vi "sftp_rename.vi"() -> ()   [LabVIEW 2017]
doc: "Illustrates how to rename a file on an SSH server."
uses:
  libssh2/libssh2_session_handshake_tcp.vi
  libssh2/libssh2_init_default.vi
  libssh2/libssh2_session_init_ex.vi
  <vilib>/Utility/tcp.llb/TCP Get Raw Net Object.vi
  libssh2/libssh2_session_handshake_socket.vi
  libssh2/libssh2_userauth_password_ex.vi
  libssh2/libssh2_sftp_rename_ex.vi
  libssh2/libssh2.lvlib
panel:
  in  "destination file":string="/"
  in  "source file":string="/"
  out "error out":errorcluster
  in  "password":string
  in  "username":string
  in  "hostname":string
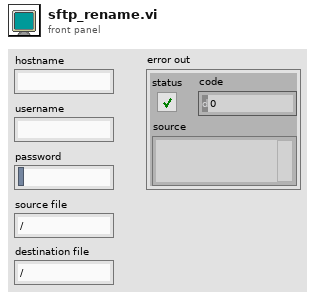
[diagram p1: front panel]
types:
  T1 = typedef "libssh2.lvlib/Session Refnum.ctl" = refnum<k1>
  T2 = typedef "libssh2.lvlib/SFTP Refnum.ctl" = refnum<k1>
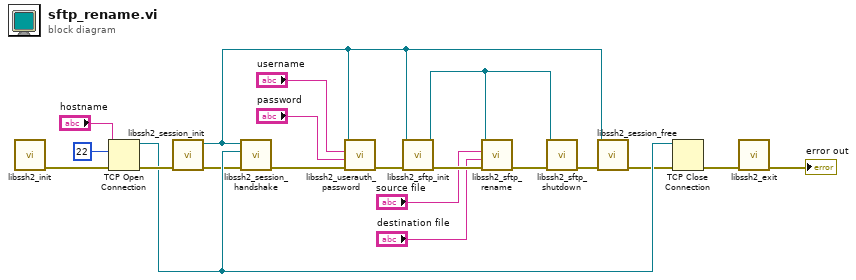
[diagram p0: block diagram]
diagram:
  n1 = call-poly "libssh2_init.vi"() -> ("error out"=w19:errorcluster)  [unwired: 11 in]
  n2 = TCP Open Connection(address="hostname", remote port or service name=u16 22, error in (no error)=w19) -> (connection ID=w17:refnum<k5>, error out=w18:errorcluster)  [unwired: 2 in]
  n3 = call "libssh2_session_init.vi"("error in (no error)"=w18) -> ("error out"=w16:errorcluster, "session"=w9:T1)  [unwired: 9 in]
  n4 = call-poly "libssh2_session_handshake.vi"("error in (no error)"=w16, "tcp connection"=w17, "session"=w9) -> ("error out"=w20:errorcluster)  [unwired: 8 in]
  n5 = call "libssh2_userauth_password.vi"("error in (no error)"=w20, "password"="password", "username"="username", "session"=w9) -> ("error out"=w13:errorcluster)  [unwired: 7 in]
  n6 = call "libssh2_sftp_init.vi"("error in (no error)"=w13, "session"=w9) -> ("error out"=w5:errorcluster, "sftp"=w4:T2)  [unwired: 8 in]
  n7 = call "libssh2_sftp_rename.vi"("error in (no error)"=w5, "destination file"="destination file", "source file"="source file", "sftp"=w4) -> ("error out"=w2:errorcluster)  [unwired: 7 in]
  n8 = call "libssh2_sftp_shutdown.vi"("error in (no error)"=w2, "sftp"=w4) -> ("error out"=w6:errorcluster)  [unwired: 9 in]
  n9 = call "libssh2_session_free.vi"("error in (no error)"=w6, "session"=w9) -> ("error out"=w8:errorcluster)  [unwired: 9 in]
  n10 = TCP Close Connection(connection ID=w17, error in (no error)=w8) -> (error out=w7:errorcluster)  [unwired: 1 in, 1 out]
  n11 = call "libssh2_exit.vi"("error in (no error)"=w7) -> ("error out"=→"error out":errorcluster)  [unwired: 10 in]
